vi "S2C_LogError.vi"(8 "Error In":errorcluster, 11 "Error Msg":string) -> (0 "Error Out":errorcluster)   [LabVIEW 2015]
doc: "Writes the error text to an error file, not to exceed 500 records. Once the limit is reached, the oldest entries will be overwritten first."
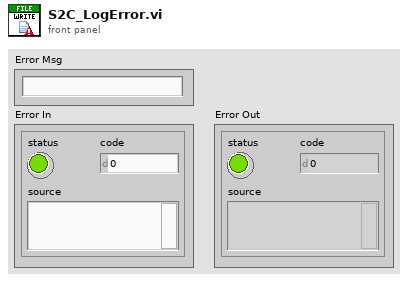
[diagram p1: front panel]
types:
  T1 = enum16{"open", "replace", "create", "open or create", "replace or create", "replace or create with confirmation"}
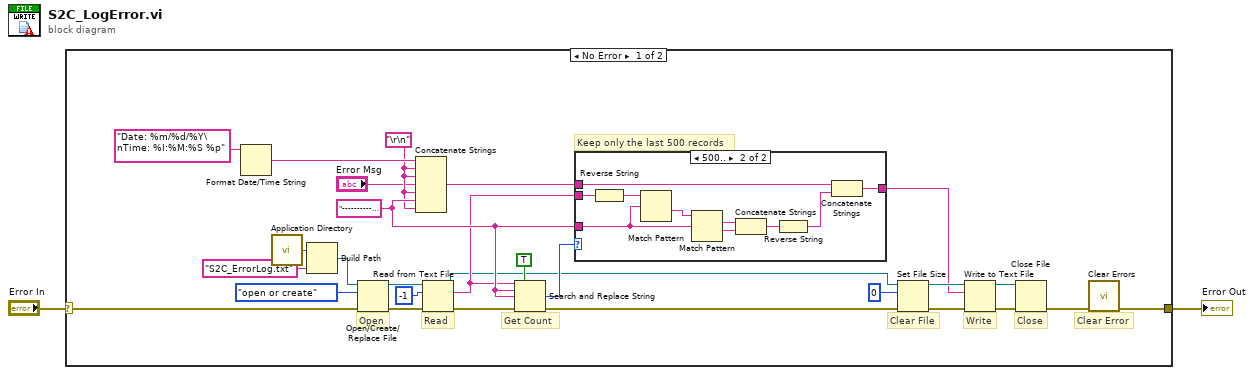
[diagram p0: block diagram]
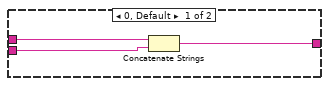
[diagram p2: hidden frame]
diagram:
  n1 = case shown="No Error" "Error In" {
    selector: "Error In" -> [w3 w44]
    tunnel: [w13 w44] -> w2
    frame No Error {
      w27 = "----------------------------------------------------------------------------------------------------"
      w5 = "\r\n"
      # "Clear Error"
      # "Get Count"
      # "Keep only the last 500 records"
      # "Write"
      # "Clear File"
      # "Close"
      # "Read"
      # "Open"
      n2 = Format Date/Time String(time format string (%c)="Date: %m/%d/%Y\nTime: %I:%M:%S %p") -> (date/time string=w15:string)  [unwired: 2 in]
      n3 = call <vilib>:"Application Directory.vi"() -> ("Application Directory"=w8:path)
      n4 = Build Path(base path=w8, name or relative path="S2C_ErrorLog.txt") -> (appended path=w6:path)
      n5 = Open/Create/Replace File(file path (use dialog)=w6, error in=w3, operation (0:open)=T1."open or create") -> (refnum out=w18:refnum<file>, error out=w19:errorcluster)  [unwired: 3 in, 1 out]
      n6 = Concatenate Strings(w15, w5, w5, "Error Msg", w5, w27, w5) -> (w11:string)
      n7 = Read from Text File(file (use dialog)=w18, count=-1, error in=w19) -> (refnum out=w10:refnum<file>, text=w26:string, error out=w25:errorcluster)  [unwired: 1 in, 1 out]
      n8 = Search and Replace String(replace all?=TRUE ("replace all? (F)"), input string=w26, search string=w27, replace string=w27, error in=w25) -> (number of replacements=w30:i32, error out=w29:errorcluster)  [unwired: 3 in, 2 out]
      n9 = case shown="500.." w30 {
        tunnel: [w31 w40] -> w12
        tunnel: w26 -> [w32 w43]
        tunnel: w27 -> [_ w37]
        tunnel: w11 -> [w33 w41]
        frame 0, Default {
          n10 = Concatenate Strings(w33, w32) -> (w31:string)
        }
        frame 500.. {
          n11 = Reverse String(1:w43) -> (0:w39:string)
          n12 = Match Pattern(string=w39, regular expression=w37) -> (after substring=w38:string)  [unwired: 1 in, 3 out]
          n13 = Match Pattern(string=w38, regular expression=w37) -> (match substring=w35:string, after substring=w36:string)  [unwired: 1 in, 2 out]
          n14 = Concatenate Strings(w35, w36) -> (w34:string)
          n15 = Reverse String(1:w34) -> (0:w42:string)
          n16 = Concatenate Strings(w41, w42) -> (w40:string)
        }
      }
      n17 = Set File Size(4:w29, 6:i64 0 ("offset (in bytes) (0)"), 7:w10) -> (0:w21:errorcluster, 3:w22:refnum<file>)
      n18 = Write to Text File(file (use dialog)=w22, text=w12, error in=w21) -> (refnum out=w24:refnum<file>, error out=w23:errorcluster)  [unwired: 1 in, 1 out]
      n19 = Close File(refnum=w24, error in=w23) -> (error out=w14:errorcluster)  [unwired: 1 out]
      n20 = call <vilib>:"Clear Errors.vi"("error in (no error)"=w14) -> ("error out"=w13:errorcluster)  [unwired: 5 in, 1 out]
    }
    frame Error {
    }
  }
  "Error Out" <- w2
